vi "Get Data Path.vi"(8 "error in":errorcluster, 11 "Data Path In":path) -> (0 "error out":errorcluster, 3 "Data Path Out":path)   [LabVIEW 2014, in "File Utilities.lvlib"]
doc: "Checks the current requested <B>Data Path In</B> to see if it exists then creates it if it does not and then creates a data log directory based on the current date."
uses:
  File Utilities.lvlib
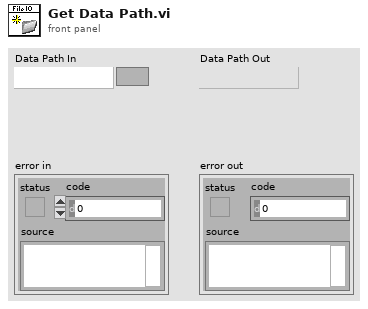
[diagram p1: front panel]
types:
  T1 = typedef "LVDateTimeRec.ctl" = cluster{"fractional second":dbl, "second":i32, "minute":i32, "hour":i32, "day of month":i32, "month":i32, "year":i32, "day of week":i32, "day of year":i32, "DST":i32}
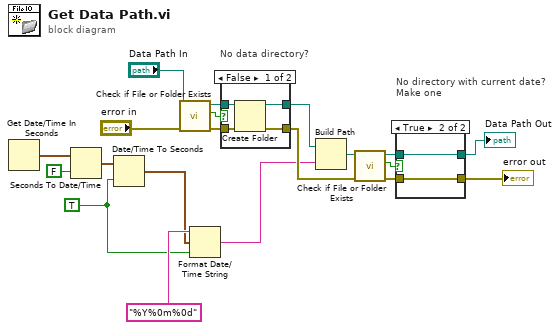
[diagram p0: block diagram]
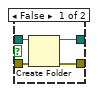
[diagram p3: hidden frame]
diagram:
  w2 = TRUE ("is UTC (F)")
  n1 = Get Date/Time In Seconds() -> (seconds since 1Jan1904=w6:timestamp)
  n2 = Seconds To Date/Time(time stamp (now)=w6, to UTC (F)=FALSE) -> (date time rec=w4:T1)
  n3 = Date/Time To Seconds(1:w2, 2:w4) -> (0:w3:timestamp)
  n4 = call <vilib>:"Check if File or Folder Exists.vi"("error in (no error)"="error in", "path"="Data Path In") -> ("error out"=w14:errorcluster, "file or folder exists?"=w16:bool, "dup path"=w15:path)  [unwired: 7 in]
  n5 = Format Date/Time String(time format string (%c)="%Y%0m%0d", seconds (now)=w3, UTC format=w2) -> (date/time string=w1:string)
  n6 = case "No data directory?" shown="False" w16 {
    tunnel: w15 -> [w23 w26]
    tunnel: [w24 w26] -> w20
    tunnel: w14 -> [w22 w25]
    tunnel: [w21 w25] -> w19
    frame False {
      n7 = Create Folder(path (use dialog)=w23, error in=w22) -> (created path=w24:path, error out=w21:errorcluster)  [unwired: 1 in, 1 out]
    }
    frame True {
    }
  }
  n8 = Build Path(base path=w20, name or relative path=w1) -> (appended path=w8:path)
  n9 = call <vilib>:"Check if File or Folder Exists.vi"("error in (no error)"=w19, "path"=w8) -> ("error out"=w11:errorcluster, "file or folder exists?"=w9:bool, "dup path"=w10:path)  [unwired: 7 in]
  n10 = case "No directory with current date?\nMake one" shown="True" w9 {
    tunnel: w10 -> [w29 w32]
    tunnel: [w30 w32] -> w13
    tunnel: w11 -> [w28 w31]
    tunnel: [w27 w31] -> w12
    frame False {
      n11 = Create Folder(path (use dialog)=w29, error in=w28) -> (created path=w30:path, error out=w27:errorcluster)  [unwired: 1 in, 1 out]
    }
    frame True {
    }
  }
  "Data Path Out" <- w13
  "error out" <- w12
